vi "Filter Gears.vi"(10 "Symbols":refnum<class "Symbol.lvclass">[](array[class]), 11 "Numbers":refnum<class "Number.lvclass">[](array[class])) -> (3 "Gears":T1(array[cluster]))   [LabVIEW 2020, in "Schema Parser.lvclass"]
uses:
  Schema Parser.lvclass
  Number/Number.lvclass
  Symbol/Symbol.lvclass
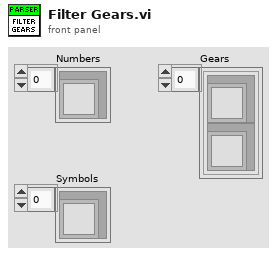
[diagram p1: front panel]
types:
  T1 = cluster{"Number":refnum<class "Number.lvclass">, "Number 2":refnum<class "Number.lvclass">}[]
  T2 = cluster{"Number":refnum<class "Number.lvclass">, "Number 2":refnum<class "Number.lvclass">}
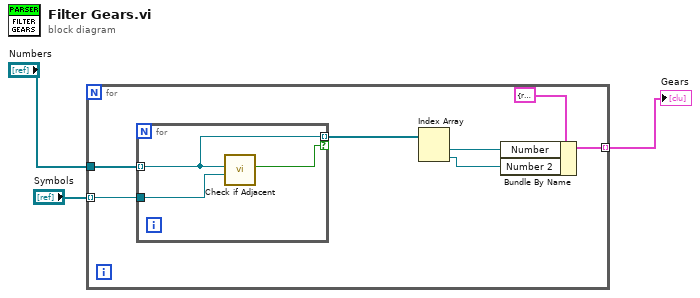
[diagram p0: block diagram]
diagram:
  n1 = for {
    tunnel: "Numbers" -> [w9]
    tunnel: "Symbols" -> [w10] mode=indexing
    tunnel: [w6] -> w1 mode=indexing
    n2 = for {
      tunnel: w9 -> [w12] mode=indexing
      tunnel: w10 -> [w13]
      tunnel: [w12] -> w8 mode=indexing if=w11
      n3 = call "Check if Adjacent.vi"("Symbol.lvclass"=w13, "Number.lvclass"=w12) -> ("Is Adjacent?"=w11:bool)  [unwired: 8 in, 1 out]
    }
    n4 = Index Array(array=w8) -> (element #1=w5:refnum<class "Number.lvclass">, element #2=w4:refnum<class "Number.lvclass">)  [unwired: 2 in]
    n5 = Bundle By Name(cluster=T2 {"Number"=refnum, "Number 2"=refnum} ("Numbers"), "Number"=w5, "Number 2"=w4) -> (w6:T2)
  }
  "Gears" <- w1
